vi "PolInit.vi"(0 "VISA resource name":refnum<visa-resource-name>, 5 "Baud Rate":T1=115200 items=["1200"=1200, "2400"=2400, "4800"=4800, "9600"=9600, "19200"=19200, "38400"=38400, "57600"=57600, "115200"=115200], 7 "Data Bits":u16=8, 9 "Parity":enum16{"None", "Odd", "Even", "Mark", "Space"}(ring), 11 "error in (no error)":errorcluster) -> (4 "VISA resource name out":refnum<visa-resource-name>, 14 "Polhemus Info":T2, 15 "error out":errorcluster)   [LabVIEW 2009]
doc: "Sets up the Polhemus Fastrak for reading. This includes setting up the COM port with the correct settings, setting up a serial port event manager to handle incoming data, and gathering information about the current Polhemus setup so that data may be read correctly."
uses:
  BaudRateSelector.ctl
  <vilib>/Instr/_visa.llb/Select Event Type.ctl
  <vilib>/Instr/_visa.llb/VISA Configure Serial Port (Instr).vi
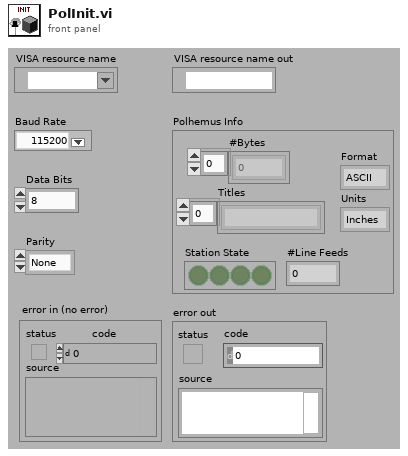
[diagram p1: front panel]
types:
  T1 = typedef "BaudRateSelector.ctl" = u32
  T2 = cluster{"#Bytes":i32[], "Titles":string[], "Format":enum16{"ASCII", "Binary"}, "Units":enum16{"Inches", "Centimeters"}, "Station State":bool[], "#Line Feeds":i32}
  T3 = typedef "Select Event Type.ctl" = u32
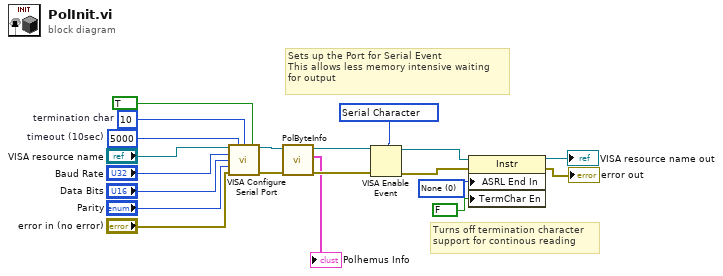
[diagram p0: block diagram]
diagram:
  w20 = T3 1073684533 items=["Service Request"=1073684491, "Trigger"=3221168138, "Clear"=1073684493, "VXI Signal"=1073684512, "VXI/VME Interrupt"=3221168161, "VXI/VME Sysfail"=1073684509, "VXI/VME Sysreset"=1073684510, "GPIB CIC"=1073684498, "GPIB Talk"=1073684499, "GPIB Listen"=1073684500, "PXI Interrupt"=1073684514, "Serial Break"=1073684515, "Serial TermChar"=1073684516, "Serial CTS"=1073684521, "Serial DSR"=1073684522, "Serial DCD"=1073684524, "Serial RI"=1073684526, "Serial Character"=1073684533, "USB Interrupt"=1073684535, "All Enabled"=1073709055] ("Event Type")
  w13 = u16 0 items=["None", "Last Bit", "TermChar"] ("Serial Settings:End Mode for Reads")
  w10 = u8 10  # termination char
  w9 = u32 5000  # timeout (10sec)
  # "Turns off termination character\nsupport for continous reading"
  # "Sets up the Port for Serial Event\nThis allows less memory intensive waiting\nfor output"
  n1 = call-poly "VISA Configure Serial Port"("VISA resource name"="VISA resource name", "timeout (10sec)"=w9, "termination char\n(0xA = '\\n' = LF)"=w10, "Enable Termination\nChar (T)"=TRUE ("Enable Termination\nChar (T)"), "baud rate (9600)"="Baud Rate", "data bits (8)"="Data Bits", "parity (0:none)"="Parity", "error in (no error)"="error in (no error)") -> ("VISA resource name out"=w7:refnum<visa-resource-name>, "error out"=w8:errorcluster)  [unwired: 6 in]
  n2 = call "PolByteInfo.vi"("error in (no error)"=w8, "VISA resource name"=w7) -> ("error out"=w16:errorcluster, "Polhemus Info"=→"Polhemus Info":T2, "VISA resource name out"=w18:refnum<visa-resource-name>)  [unwired: 5 in]
  n3 = VISA Enable Event(8:w16, 10:w20, 11:w18) -> (0:w17:errorcluster, 3:w19:refnum<visa-resource-name>)  [unwired: 1 in]
  n4 = property class="Instr"(reference=w19, error in=w17, "ASRL End In"=w13, "TermChar En"=FALSE ("Message Based Settings:Termination Character Enable")) -> (reference out=→"VISA resource name out":refnum<visa-resource-name>, error out=→"error out":errorcluster)
